vi "GetAuxSequence.vi"(8 "error in (no error)":errorcluster, 11 "Compiler Settings":T1={"Python Path"=path "", "Main File"="mainscript.py", "Meta File"="metascript.txt", "Aux File"="auxscript.py", "Pre File"="metascript.txt"}) -> (0 "error out":errorcluster, 3 "Aux Pulse":T2)   [LabVIEW 2019]
uses:
  PulseControl.ctl
  Compiler/Params.ctl
  PulseCompiler/CompilerSettings.ctl
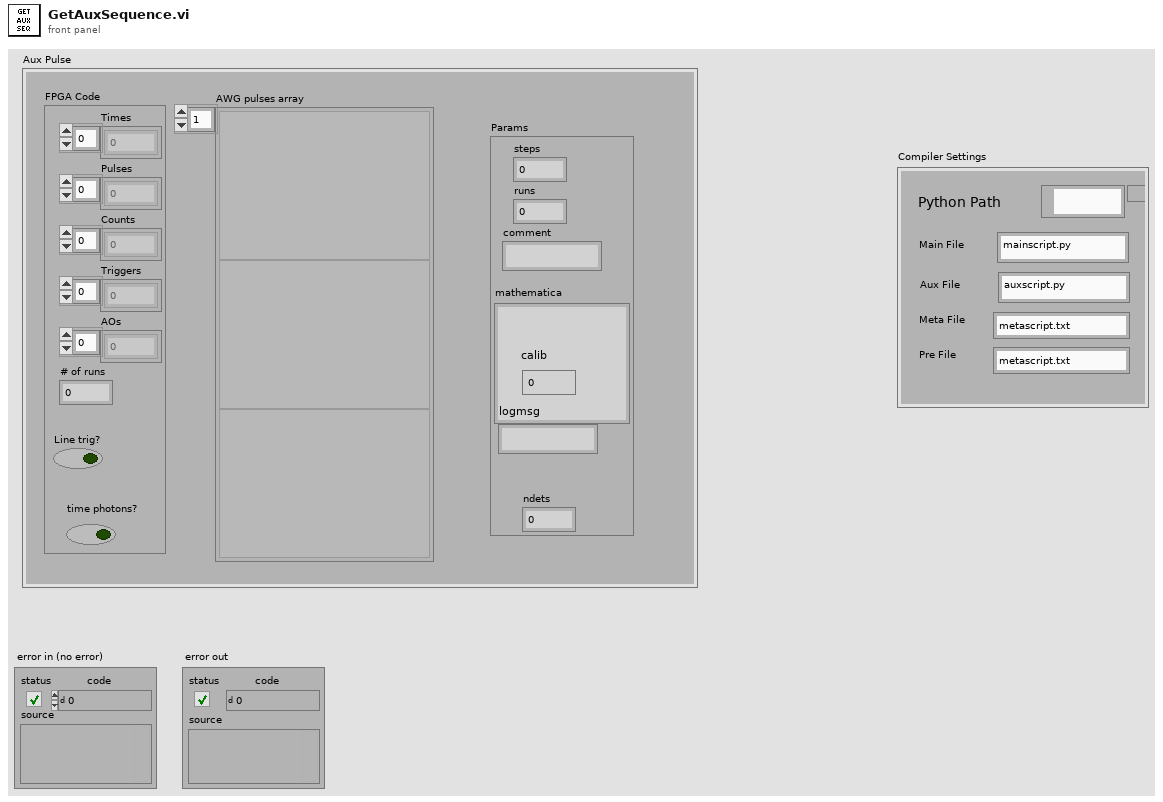
[diagram p1: front panel]
types:
  T1 = typedef "CompilerSettings.ctl" = cluster{"Python Path":path, "Main File":string, "Meta File":string, "Aux File":string, "Pre File":string}
  T2 = typedef "PulseControl.ctl" = cluster{"FPGA Code":cluster{"Times":u32[], "Pulses":u64[], "Counts":u8[], "Triggers":u8[], "AOs":u8[], "# of runs":i32, "Line trig?":bool, "time photons?":bool}, "AWG pulses array":variant[], "Params":T3}
  T3 = typedef "Params.ctl" = cluster{"steps":i16, "runs":i16, "comment":string, "mathematica":string, "calib":i8, "logmsg":string, "ndets":i16}
  T4 = typedef "SinglePulse.ctl" = cluster{"enabled":bool, "string":string, "time":dbl, "step":dbl, "dio":dbl, "count":dbl, "trigger":dbl, "AO":dbl}
  T5 = cluster{u32[], dbl[], "Count":dbl[], dbl[], dbl[], "# of runs":i32, "Line trig":bool, "save photon times":bool}
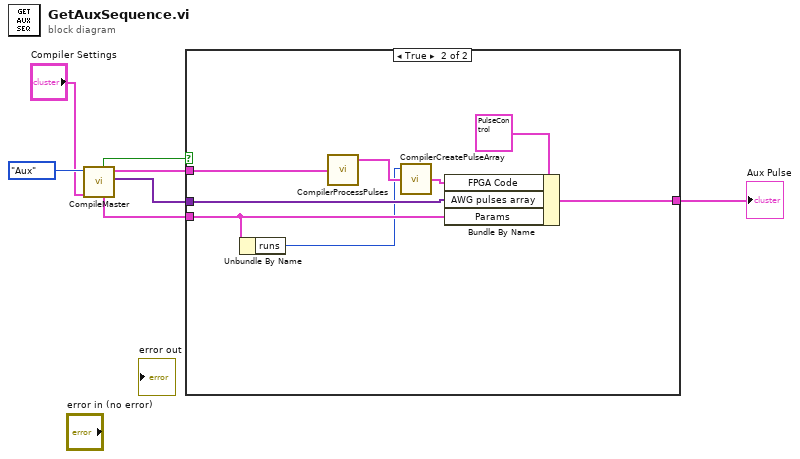
[diagram p0: block diagram]
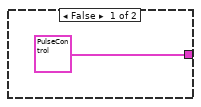
[diagram p2: hidden frame]
diagram:
  n1 = call "CompileMaster.vi"("Type"=enum16{"Meta", "Aux", "Main"}."Aux" ("Enum"), "Compiler Settings"="Compiler Settings") -> ("CompileSuccess?"=w7:bool, "Params"=w6:T3, "PulseList"=w4:T4[], "RF Array"=w3:variant[])  [unwired: 2 in, 2 out]
  n2 = case shown="True" w7 {
    tunnel: [T2 {"FPGA Code"={"Times"=[], "Pulses"=[], "Counts"=[], "Triggers"=[], "AOs"=[], "# of runs"=0, "Line trig?"=FALSE, "time photons?"=FALSE}, "AWG pulses array"=[], "Params"={"steps"=0, "runs"=0, "comment"="", "mathematica"="", "calib"=0, "logmsg"="", "ndets"=0}} ("Pulse") w16] -> w2
    tunnel: w3 -> [_ w15]
    tunnel: w4 -> [_ w12]
    tunnel: w6 -> [_ w11]
    frame False {
    }
    frame True {
      n3 = Unbundle By Name(w11) -> ("runs"=w10:i16)
      n4 = call "CompilerProcessPulses.vi"("Pulse Seq In"=w12) -> ("Pulse Seq Out"=w14:T4[])  [unwired: 2 out]
      n5 = call "CompilerCreatePulseArray.vi"("Pulse Seq In"=w14, "runs"=w10) -> ("Pulse Seq Out"=w13:T5)  [unwired: 1 in]
      n6 = Bundle By Name(cluster=T2 {"FPGA Code"={"Times"=[], "Pulses"=[], "Counts"=[], "Triggers"=[], "AOs"=[], "# of runs"=0, "Line trig?"=FALSE, "time photons?"=FALSE}, "AWG pulses array"=[], "Params"={"steps"=0, "runs"=0, "comment"="", "mathematica"="", "calib"=0, "logmsg"="", "ndets"=0}} ("Aux Pulse 2"), "FPGA Code"=w13, "AWG pulses array"=w15, "Params"=w11) -> (w16:T2)
    }
  }
  "Aux Pulse" <- w2
